vi "Namen aus Tabelle ersetzen.vi"(8 "Fehler (Eingang, kein Fehler)":errorcluster, 9 "Regulärer Ausdruck":string, 10 "Sprachauswahl":u16, 11 "Tabelle":string[][](array[string])) -> (0 "Fehler (Ausgang)":errorcluster, 2 "found":bool, 3 "Übersetzung":string)   [LabVIEW 2020, in "Sprachverwaltung.lvlib"]
uses:
  Sprachverwaltung.lvlib
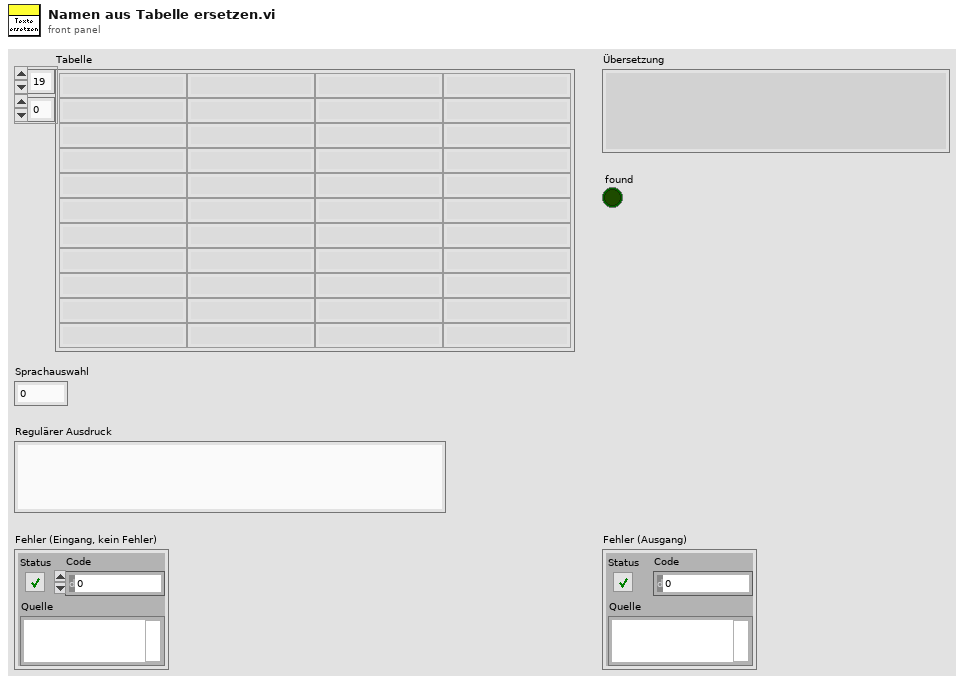
[diagram p1: front panel]
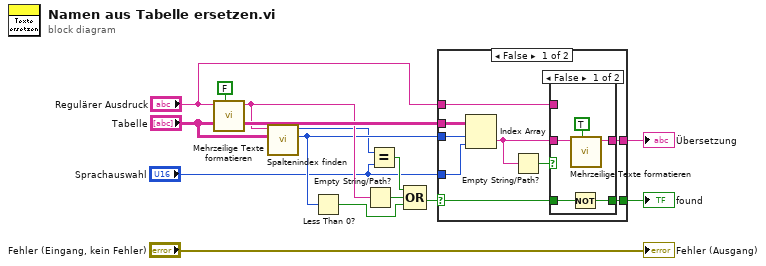
[diagram p0: block diagram]
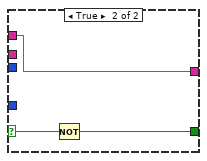
[diagram p3: hidden frame]
diagram:
  n1 = call "Mehrzeilige Texte formatieren.vi"("Zurück formatieren"=FALSE, "string"="Regulärer Ausdruck") -> ("result string"=w10:string)  [unwired: 9 in]
  n2 = call "Spaltenindex finden.vi"("Tabelle"="Tabelle", "Regulärer Ausdruck"=w10) -> ("Tab Zeile"=w5:i32, "Tab Spalte"=w2:i32)  [unwired: 8 in]
  n3 = Less Than 0?(x=w5) -> (x < 0?=w6:bool)
  n4 = Empty String/Path?(string/path=w10) -> (empty?=w13:bool)
  n5 = Equal?(x=w2, y="Sprachauswahl") -> (x = y?=w4:bool)
  n6 = Compound Arithmetic op=OR ("Mehrfacharithmetik")(w4, w13, w6) -> (w14:bool)
  n7 = case shown="False" w14 {
    selector: w14 -> [w20 w32]
    tunnel: [w21 w33] -> w8
    tunnel: "Sprachauswahl" -> [w23 _]
    tunnel: "Tabelle" -> [w22 _]
    tunnel: "Regulärer Ausdruck" -> [w15 w33]
    tunnel: [w18 w31] -> w7
    tunnel: w5 -> [w19 _]
    frame False {
      n8 = Index Array(array=w22, index (row)=w19, index (col)=w23) -> (element=w17:string)
      n9 = Empty String/Path?(string/path=w17) -> (empty?=w16:bool)
      n10 = case shown="False" w16 {
        tunnel: w17 -> [w27 _]
        tunnel: [w26 w29] -> w21
        tunnel: w20 -> [w25 w30]
        tunnel: [w24 w30] -> w18
        tunnel: w15 -> [_ w29]
        frame False {
          n11 = Not(x=w25) -> (.not. x?=w24:bool)
          n12 = call "Mehrzeilige Texte formatieren.vi"("Zurück formatieren"=TRUE, "string"=w27) -> ("result string"=w26:string)  [unwired: 9 in]
        }
        frame True {
        }
      }
    }
    frame True {
      n13 = Not(x=w32) -> (.not. x?=w31:bool)
    }
  }
  "Übersetzung" <- w8
  "found" <- w7
  "Fehler (Ausgang)" <- "Fehler (Eingang, kein Fehler)"
